vi "Day 1.1 - Sweep for increasing measurments.vi"(11 "input":i32[](array[numeric])) -> (3 "output":i16)   [LabVIEW 2021]
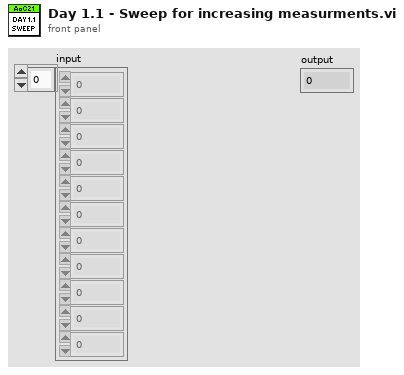
[diagram p1: front panel]
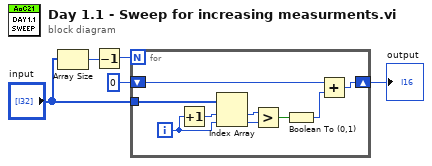
[diagram p0: block diagram]
diagram:
  n1 = Array Size(array="input") -> (size(s)=w3:i32)
  n2 = Decrement(x=w3) -> (x-1=w4:i32)
  n3 = for {
    N: w4 -> [_]
    tunnel: "input" -> [w12]
    shift-right: [w10] -> w5
    shift-left: i16 0 -> [w11]
    i -> [w6]
    n4 = Increment(x=w6) -> (x+1=w7:i32)
    n5 = Index Array(array=w12, index #1=w7, index #2=w6) -> (element #1=w14:i32, element #2=w13:i32)
    n6 = Greater?(x=w14, y=w13) -> (0:w9:bool)
    n7 = Boolean To (0,1)(Boolean=w9) -> (0, 1=w8:i16)
    n8 = Add(x=w11, y=w8) -> (x+y=w10:i16)
  }
  "output" <- w5
